vi "Add Row to Configuration Listbox.vi"(7 "Plot Colour Box":u32, 8 "error in":errorcluster, 9 "Descriptive Name":string, 10 "Data Source Selector Ref":refnum<vi>, 11 "Configuraiton Listbox Ref":refnum<vi>) -> (0 "error out":errorcluster)   [LabVIEW 2017, in "DTacq Plot Display Library.lvlib"]
uses:
  DTacq Plot Display Library.lvlib
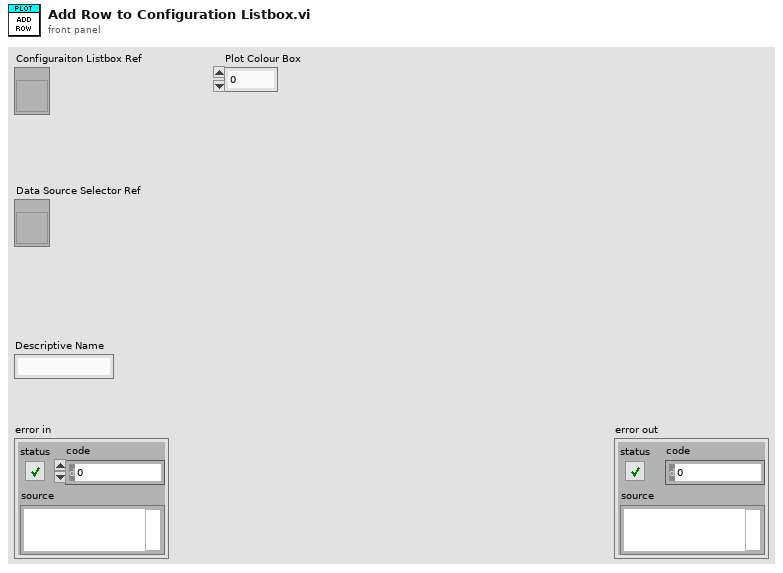
[diagram p1: front panel]
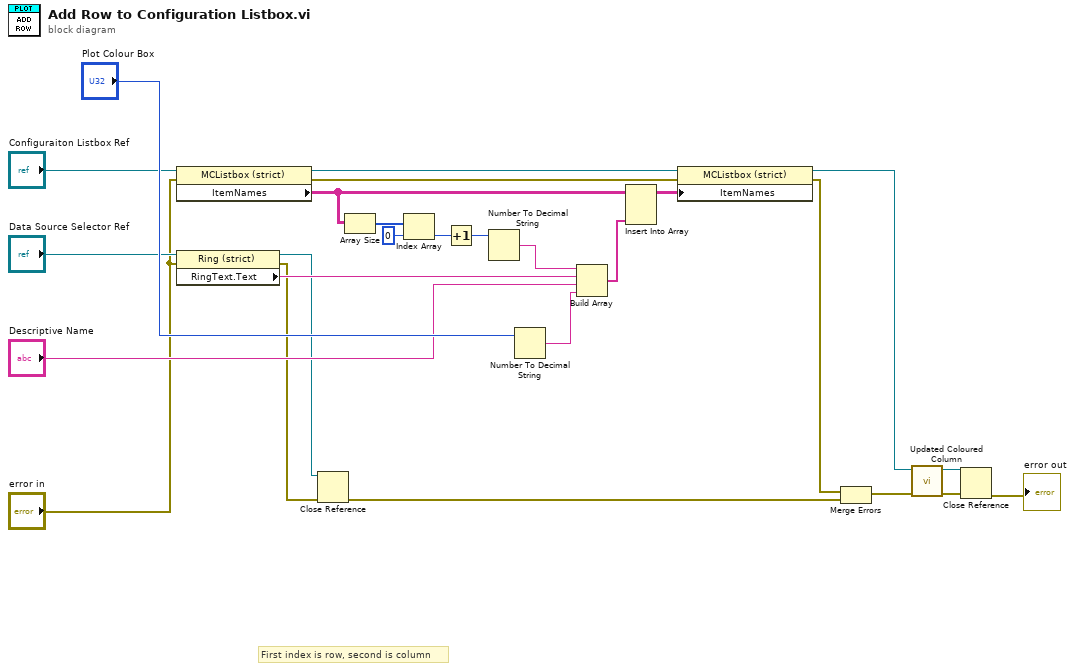
[diagram p0: block diagram]
diagram:
  # "First index is row, second is column"
  n1 = property class="MCListbox (strict)"(reference="Configuraiton Listbox Ref", error in="error in") -> (reference out=w17:refnum<vi>, error out=w11:errorcluster, "ItemNames"=w18:string[][])
  n2 = property class="Ring (strict)"(reference="Data Source Selector Ref", error in="error in") -> (reference out=w7:refnum<vi>, error out=w8:errorcluster, "RingText.Text"=w14:string)
  n3 = Close Reference(reference=w7, error in (no error)=w8) -> (error out=w6:errorcluster)
  n4 = Array Size(array=w18) -> (size(s)=w19:i32[])
  n5 = Index Array(array=w19, index=0) -> (element=w24:i32)
  n6 = Increment(x=w24) -> (x+1=w21:i32)
  n7 = Number To Decimal String(number=w21) -> (decimal integer string=w22:string)  [unwired: 1 in]
  n8 = Number To Decimal String(number="Plot Colour Box") -> (decimal integer string=w25:string)  [unwired: 1 in]
  n9 = Build Array(w22, w14, "Descriptive Name", w25) -> (w15:string[])
  n10 = Insert Into Array(array=w18, new element=w15) -> (w16:string[][])  [unwired: 2 in]
  n11 = property class="MCListbox (strict)"(reference=w17, error in=w11, "ItemNames"=w16) -> (reference out=w5:refnum<vi>, error out=w4:errorcluster)
  n12 = Merge Errors(w4, w6) -> (w3:errorcluster)
  n13 = call "Updated Coloured Column.vi"("error in"=w3, "MulticolumnListbox in"=w5) -> ("error out"=w2:errorcluster, "MulticolumnListbox Out"=w1:refnum<vi>)  [unwired: 8 in]
  n14 = Close Reference(reference=w1, error in (no error)=w2) -> (error out=→"error out":errorcluster)
